vi "Pop-up window.vi"() -> ()   [LabVIEW 2015]
panel:
  in  "Help":bool
  in  "Num. Ind. 1":dbl format="%#.4g"
  in  "Button 1":bool
  out "Graph":T1(graph)
  in  "Num. Ind. 4":dbl format="%#.4g"
  in  "Num. Ind. 3":dbl format="%#.4g"
  in  "Button 4":bool
  in  "Button 3":bool
  in  "Button 2":bool
  in  "stop":bool
  in  "Table":bool
  in  "D(U)":bool
  in  "C(U)":bool
  in  "Площадь контакта, кв.мм 2":dbl format="%#.4g"
  in  "Num. Ind. 2":dbl format="%#.4g"
  in  "X(N)":bool
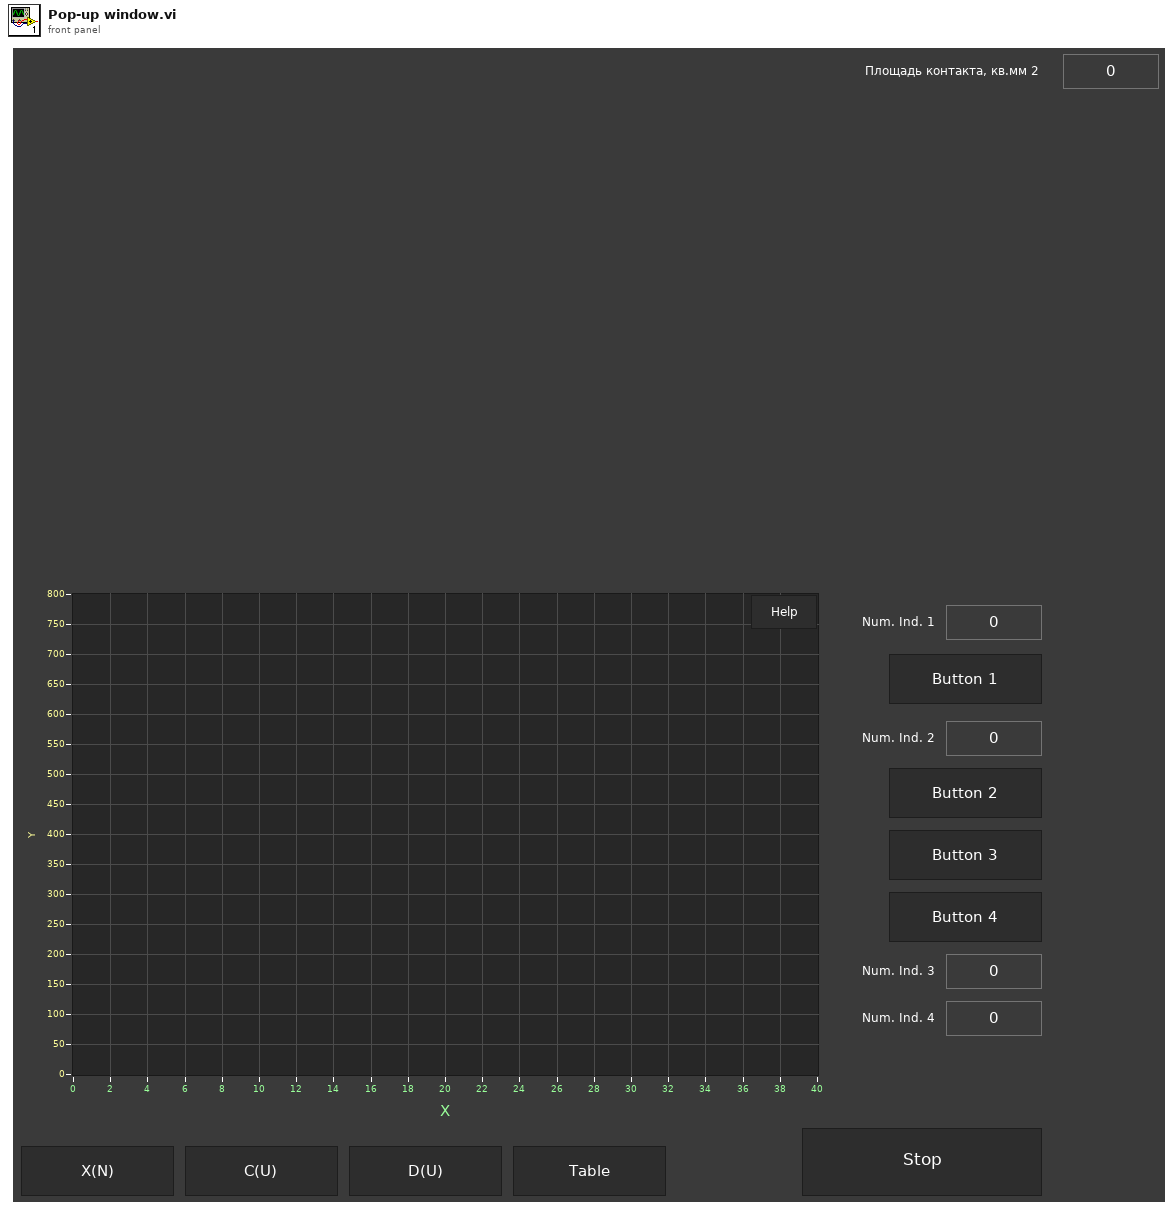
[diagram p1: front panel]
types:
  T1 = cluster{"Frequency Points Array":dbl[], "Data":dbl[]}[]
  T2 = cluster{"Mouse queue":refnum<queue>, "Stop queue":refnum<queue>}
  T3 = cluster{"Graph":refnum<vi>, "X(N)":refnum<vi>, "C(U)":refnum<vi>, "D(U)":refnum<vi>, "Table":refnum<vi>, "stop":refnum<vi>, "Button 1":refnum<vi>, "Button 2":refnum<vi>, "Button 3":refnum<vi>, "Button 4":refnum<vi>, "Num. Ind. 1":refnum<vi>, "Num. Ind. 2":refnum<vi>, "Num. Ind. 3":refnum<vi>, "Num. Ind. 4":refnum<vi>, "Help":refnum<vi>, "This VI":refnum<vi>, "Queues":cluster{"Mouse queue":refnum<queue>, "Stop queue":refnum<queue>}}
  T4 = typedef "LVRectTypeDef.ctl" = cluster{"Left":i16, "Top":i16, "Right":i16, "Bottom":i16}
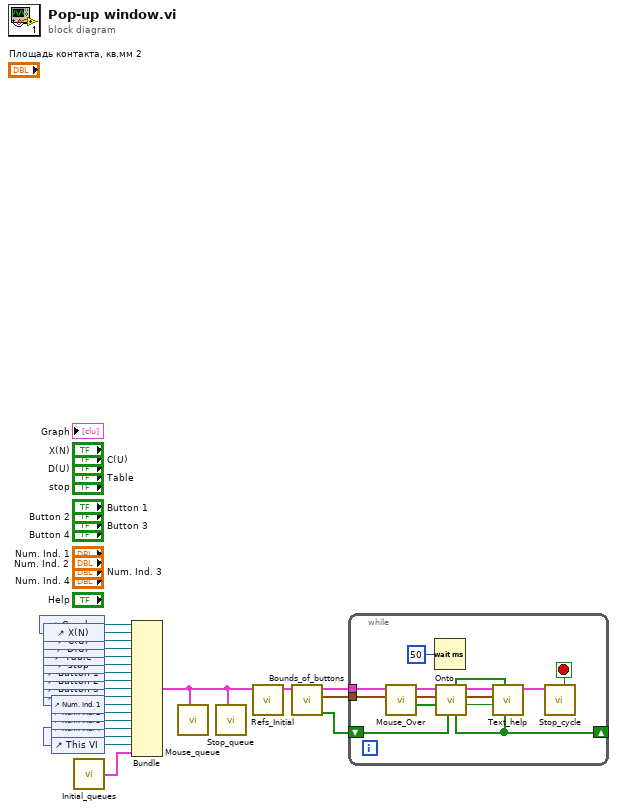
[diagram p0: block diagram]
diagram:
  n1 = control-ref of="Graph"() -> (w18:refnum<vi>)
  n2 = control-ref of="X(N)"() -> (w22:refnum<vi>)
  n3 = control-ref of="C(U)"() -> (w21:refnum<vi>)
  n4 = control-ref of="D(U)"() -> (w20:refnum<vi>)
  n5 = control-ref of="Table"() -> (w19:refnum<vi>)
  n6 = control-ref of="stop"() -> (w17:refnum<vi>)
  n7 = control-ref of="Button 1"() -> (w16:refnum<vi>)
  n8 = control-ref of="Button 2"() -> (w15:refnum<vi>)
  n9 = control-ref of="Button 3"() -> (w14:refnum<vi>)
  n10 = control-ref of="Button 4"() -> (w13:refnum<vi>)
  n11 = control-ref of="Help"() -> (w8:refnum<vi>)
  n12 = control-ref of="Num. Ind. 1"() -> (w12:refnum<vi>)
  n13 = control-ref of="Num. Ind. 2"() -> (w11:refnum<vi>)
  n14 = control-ref of="Num. Ind. 3"() -> (w10:refnum<vi>)
  n15 = control-ref of="Num. Ind. 4"() -> (w9:refnum<vi>)
  n16 = control-ref of="This VI"() -> (w7:refnum<vi>)
  n17 = call "Initial_queues.vi"() -> ("Queues"=w6:T2)  [unwired: 1 in]
  n18 = Bundle("Graph"=w18, "X(N)"=w22, "C(U)"=w21, "D(U)"=w20, "Table"=w19, "stop"=w17, "Button 1"=w16, "Button 2"=w15, "Button 3"=w14, "Button 4"=w13, "Num. Ind. 1"=w12, "Num. Ind. 2"=w11, "Num. Ind. 3"=w10, "Num. Ind. 4"=w9, "Help"=w8, "This VI"=w7, "Queues"=w6) -> (w1:T3)  [unwired: 1 in]
  n19 = call "Mouse_queue.vi"("Refs cluster In"=w1) -> ()  [unwired: 11 in]
  n20 = call "Stop_queue.vi"("Refs cluster In"=w1) -> ()  [unwired: 11 in]
  n21 = call "Refs_Initial.vi"("Refs cluster In"=w1) -> ("Refs cluster Out"=w5:T3)  [unwired: 6 in]
  n22 = call "Bounds_of_buttons.vi"("Refs cluster In"=w5) -> ("False Array"=w3:bool[], "Bounds"=w2:T4[], "Refs cluster Out"=w4:T3)  [unwired: 8 in]
  n23 = while {
    shift-right: [w25] -> _
    shift-left: w3 -> [w30]
    tunnel: w4 -> [w33]
    tunnel: w2 -> [w28]
    stop <- w23 stop-if-true
    n24 = call "Mouse_Over.vi"("Bounds"=w28, "Refs cluster In"=w33) -> ("Onto"=w32:bool[], "Refs cluster Out"=w31:T3)  [unwired: 8 in]
    n25 = Wait (ms)(milliseconds to wait=u32 50) -> ()  [unwired: 1 out]
    n26 = call "Onto.vi"("Old"=w30, "Onto"=w32, "Refs cluster In"=w31) -> ("Changed"=w29:bool, "Refs cluster Out"=w27:T3, "New"=w25:bool[], "Trigger array"=w26:bool[])  [unwired: 5 in]
    n27 = call "Text_help.vi"("Onto"=w25, "Trigger Array"=w26, "Changed"=w29, "Bounds"=w28, "Refs cluster In"=w27) -> ("Refs cluster Out"=w24:T3)  [unwired: 6 in]
    n28 = call "Stop_cycle.vi"("Refs cluster In"=w24) -> ("Stop?"=w23:bool)  [unwired: 10 in]
  }
